vi "GPS PositionFixStateChange Event Example.vi"() -> ()   [LabVIEW 2012, in "Phidget GPS.lvlib"]
uses:
  <instrlib>/Phidgets/Phidget GPS/Phidget GPS.lvlib
  <instrlib>/Phidgets/Phidget GPS/Public/GPSStart.vi
  <instrlib>/Phidgets/Phidget GPS/Public/GPSClose.vi
  <instrlib>/Phidgets/Phidget Common/Phidget Common.lvlib
panel:
  out "FixState":bool
  in  "stop":bool
  out "Serial Number Return":i32
  in  "Device Info":T1={"Serial Number"=-1, "Channel"=0, "Port"=0}
  out "error out":errorcluster
  # "Be sure to use this stop button to stop the program.\nIf you use the \"Abort Execution\" button, you will\nneed to use PhidgetResetLibrary.vi or restart Labview \nin order for any Phidgets to work."
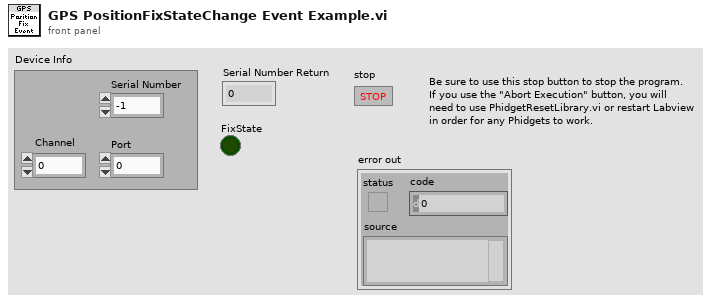
[diagram p1: front panel]
types:
  T1 = cluster{"Serial Number":i32, "Channel":i32, "Port":i32}
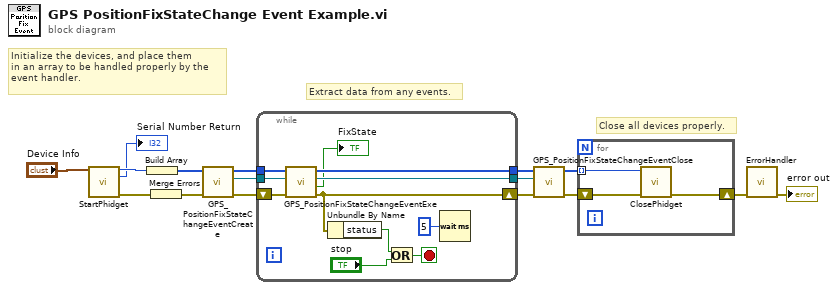
[diagram p0: block diagram]
diagram:
  # "Close all devices properly."
  # "Extract data from any events."
  # "Initialize the devices, and place them\nin an array to be handled properly by the\nevent handler."
  n1 = call-poly <instrlib>:"StartPhidget.vi"("Device Info"="Device Info") -> ("Phidget ID"=w5:u64, "Serial Number Return"=→"Serial Number Return":i32, "error out"=w2:errorcluster)  [unwired: 11 in, 1 out]
  n2 = Build Array(w5) -> (w16:u64[])
  n3 = Merge Errors(w2) -> (w7:errorcluster)
  n4 = call <instrlib>:"GPS_PositionFixStateChangeEventCreate.vi"("error in (no error)"=w7, "Devices In"=w16) -> ("error out"=w9:errorcluster, "Event Registration Refnum"=w14:refnum<event-registration>, "Devices Out"=w15:u64[])  [unwired: 7 in]
  n5 = while {
    tunnel: w15 -> [w27]
    tunnel: w14 -> [w22]
    tunnel: [w26] -> w11
    shift-right: [w21] -> w10
    shift-left: w9 -> [w25]
    tunnel: [w23] -> w3
    stop <- w20 stop-if-true
    n6 = call <instrlib>:"GPS_PositionFixStateChangeEventExe.vi"("error in (no error)"=w25, "Event Registration Refnum In"=w22, "Devices In"=w27) -> ("error out"=w21:errorcluster, "FixState"=→"FixState":bool, "Event Registration Refnum Out"=w26:refnum<event-registration>, "Devices Out"=w23:u64[])  [unwired: 2 in, 3 out]
    n7 = Unbundle By Name(w21) -> ("status"=w18:bool)
    n8 = Or(x=w18, y="stop") -> (x .or. y?=w20:bool)
    n9 = Wait (ms)(milliseconds to wait=u32 5) -> ()  [unwired: 1 out]
  }
  n10 = call <instrlib>:"GPS_PositionFixStateChangeEventClose.vi"("error in (no error)"=w10, "Event Registration Refnum In"=w11, "Devices In"=w3) -> ("error out"=w6:errorcluster, "Devices Out"=w4:u64[])  [unwired: 7 in]
  n11 = for {
    tunnel: w4 -> [w28] mode=indexing
    shift-right: [w30] -> w13
    shift-left: w6 -> [w29]
    n12 = call-poly <instrlib>:"ClosePhidget.vi"("error in"=w29, "Device In"=w28) -> ("error out"=w30:errorcluster)  [unwired: 9 in]
  }
  n13 = call <instrlib>:"ErrorHandler.vi"("error in"=w13) -> ("error out"=→"error out":errorcluster)  [unwired: 9 in, 1 out]
